vi "CalculateNextValue.vi"(0 "Target a 2":dbl, 1 "Channel a source value":dbl, 2 "Ch a sweep rate units/min":dbl, 3 "time between points, sec":dbl, 4 "Source a":T1) -> (5 "Target a":dbl, 6 "Boolean":bool)   [LabVIEW 2021]
uses:
  controls/Source.ctl
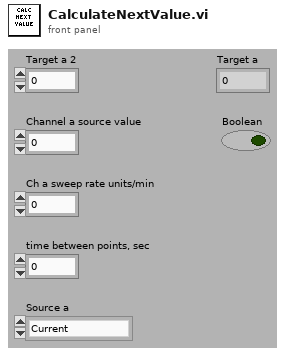
[diagram p1: front panel]
types:
  T1 = typedef "Source.ctl" = enum16{"Current", "Voltage"}
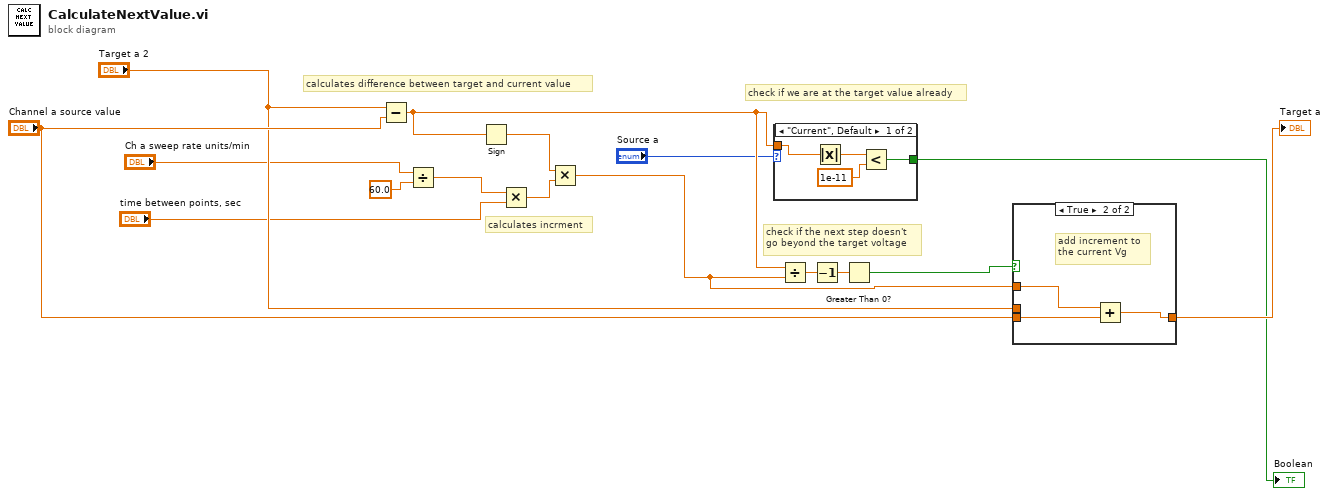
[diagram p0: block diagram]
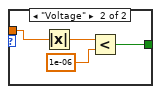
[diagram p3: hidden frame]
diagram:
  # "check if the next step doesn't\ngo beyond the target voltage"
  # "check if we are at the target value already"
  # "calculates incrment"
  # "calculates difference between target and current value"
  n1 = Subtract(x="Target a 2", y="Channel a source value") -> (x-y=w11:dbl)
  n2 = Divide(x="Ch a sweep rate units/min", y=60.0) -> (x/y=w4:dbl)
  n3 = Sign(1:w11) -> (0:w5:dbl)
  n4 = Multiply(x=w4, y="time between points, sec") -> (x*y=w6:dbl)
  n5 = Multiply(x=w5, y=w6) -> (x*y=w14:dbl)
  n6 = case shown="\"Current\", Default" "Source a" {
    tunnel: w11 -> [w18 w22]
    tunnel: [w17 w21] -> w8
    frame "Current", Default {
      n7 = Absolute Value(x=w18) -> (abs(x)=w20:dbl)
      n8 = Less?(x=w20, y=1e-11) -> (x < y?=w17:bool)
    }
    frame "Voltage" {
      n9 = Absolute Value(x=w22) -> (abs(x)=w24:dbl)
      n10 = Less?(x=w24, y=1e-06) -> (x < y?=w21:bool)
    }
  }
  "Boolean" <- w8
  n11 = Divide(x=w11, y=w14) -> (x/y=w10:dbl)
  n12 = Decrement(x=w10) -> (x-1=w9:dbl)
  n13 = Greater Than 0?(x=w9) -> (x > 0?=w12:bool)
  n14 = case shown="True" w12 {
    tunnel: "Channel a source value" -> [_ w28]
    tunnel: w14 -> [_ w27]
    tunnel: [w25 w26] -> w16
    tunnel: "Target a 2" -> [w25 _]
    frame False {
      # "if next step is too long\nuse target voltage"
    }
    frame True {
      # "add increment to\nthe current Vg"
      n15 = Add(x=w27, y=w28) -> (x+y=w26:dbl)
    }
  }
  "Target a" <- w16
